vi "Write Num or Array.vi"(8 "error in (no error)":errorcluster, 10 "Ctl Refnum":refnum<vi>, 11 "Worksheet Reference":refnum<k7>) -> (0 "error out":errorcluster)   [LabVIEW 2011, in "Design Server.lvlib"]
uses:
  Design Server.lvlib
panel:
  in  "1D Array":dbl[](array[numeric]) format="%.2f"
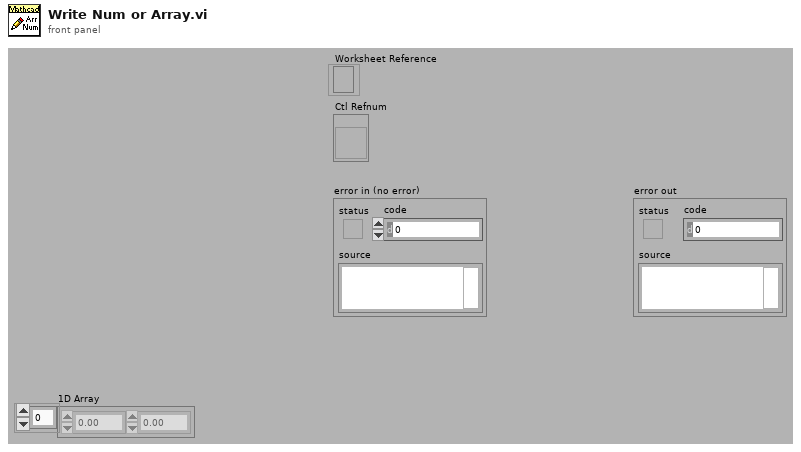
[diagram p1: front panel]
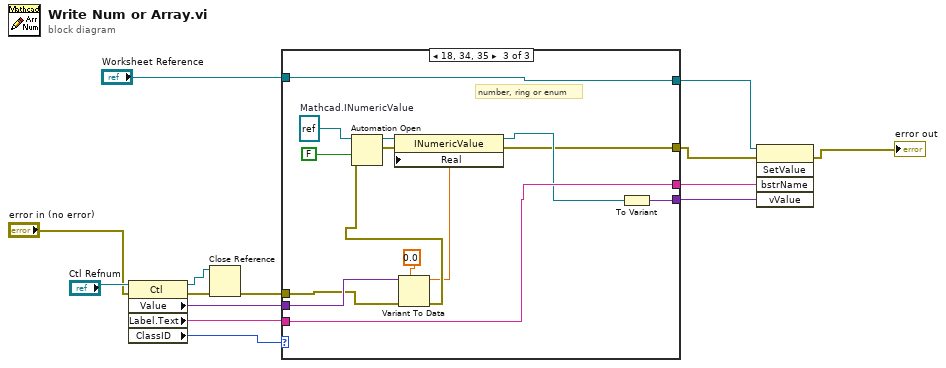
[diagram p0: block diagram]
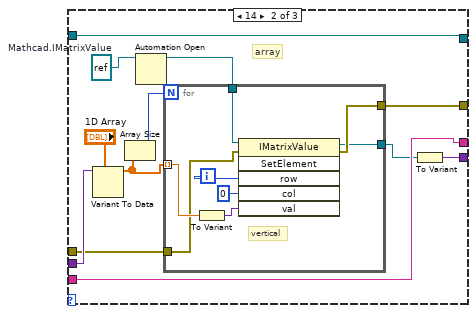
[diagram p3: hidden frame]
diagram:
  n1 = property class="Ctl"(reference="Ctl Refnum", error in="error in (no error)") -> (reference out=w10:refnum<vi>, error out=w9:errorcluster, "Value"=w14:variant, "Label.Text"=w7:string, "ClassID"=w11:u32)
  n2 = Close Reference(reference=w10, error in (no error)=w9) -> (error out=w8:errorcluster)
  n3 = case shown="18, 34, 35" w11 {
    tunnel: w8 -> [w15 w23 w42]
    tunnel: w14 -> [_ w27 w46]
    tunnel: [w15 w17 w36] -> w4
    tunnel: w7 -> [_ w18 w38]
    tunnel: "Worksheet Reference" -> [_ w20 w40]
    tunnel: [_ w20 w40] -> w5
    tunnel: [_ w19 w39] -> w3
    tunnel: [_ w18 w38] -> w2
    frame 0, Default {
    }
    frame 14 {
      w22 = refnum<k7> refnum  # Mathcad.IMatrixValue
      # "array"
      n4 = Variant To Data(type="1D Array", Variant=w27) -> (data=w24:dbl[])  [unwired: 1 in, 1 out]
      n5 = Array Size(array=w24) -> (size(s)=w25:i32)
      n6 = Automation Open(Automation Refnum=w22) -> (Automation Refnum=w21:refnum<k7>)  [unwired: 3 in, 1 out]
      n7 = for {
        N: w25 -> [_]
        tunnel: w24 -> [w32] mode=indexing
        tunnel: w21 -> [w35]
        tunnel: w23 -> [w30]
        tunnel: [w29] -> w17
        tunnel: [w28] -> w16
        i -> [w33]
        # "vertical"
        n8 = To Variant(anything=w32) -> (Variant=w31:variant)
        n9 = invoke class="IMatrixValue" method="SetElement"(reference=w35, error in=w30, "row"=w33, "col"=0, "val"=w31) -> (reference out=w28:refnum<k7>, error out=w29:errorcluster)  [unwired: 1 in, 4 out]
      }
      n10 = To Variant(anything=w16) -> (Variant=w19:variant)
    }
    frame 18, 34, 35 {
      w45 = refnum<k7> refnum  # Mathcad.INumericValue
      # "number, ring or enum"
      n11 = Variant To Data(error in=w42, type=0.0, Variant=w46) -> (data=w41:dbl, error out=w43:errorcluster)
      n12 = Automation Open(error in (no error)=w43, Automation Refnum=w45, 9:FALSE ("open new instance")) -> (Automation Refnum=w48:refnum<k7>, error out=w47:errorcluster)  [unwired: 1 in]
      n13 = property class="INumericValue"(reference=w48, error in=w47, "Real"=w41) -> (reference out=w37:refnum<k7>, error out=w36:errorcluster)
      n14 = To Variant(anything=w37) -> (Variant=w39:variant)
    }
  }
  n15 = invoke method="SetValue"(reference=w5, error in=w4, "bstrName"=w2, "vValue"=w3) -> (error out=→"error out":errorcluster)  [unwired: 1 in, 4 out]
